vi "PH_PowerUnit_BaseClass.set modified data.vi"(0 "i ref in":refnum<vi>, 2 "i attribute":T1={"Constructor finished"=FALSE, "PU"={"In use"=FALSE, "Service ID in use"=-1, "GUI Ref"=refnum}, "Enabling"={"State"=0, "GUI Ref"=refnum}, "Timing"={"Last Shot"=0.0, "Time between Shots [Sec]"=30.0, "Waiting Time over?"=FALSE, "Service ID Waiting Time"=-1, "GUI Ref"=refnum, "Instance"={"Status"=0, "linked?"=FALSE, "GUI Ref"=refnum}}, "Sequencer"={"SM State"="N/A", "GUI Ref"=refnum, "linked"=FALSE}, "Subscribed Trendmssgs"=[], "PP PU"=enum."no Info", "Default Voltage (V)"=0.0, "GUI Refs"={"Delete Inst"=refnum, "State TO SM"=refnum, "State SM"=refnum, "Fire"=refnum}, "PSDB data"={"Shot Voltage [V]"=-1.0, "State TO SM"=enum.".", "Write 2 early"=FALSE}, "State TO SM"=enum."."} {"Subscribed Trendmssgs"."Shot Condition" items=["no info", "off/false/out", "on/true/in", "Failure", "Alarm", "Status 1", "Status 2", "Status 3"]; "Subscribed Trendmssgs"."Status" items=["no info", "off/false/out", "on/true/in", "Failure", "Alarm", "Status 1", "Status 2", "Status 3"]; "Timing"."Instance"."Status" items=["no info", "off/false/out", "on/true/in", "Failure", "Alarm", "Status 1", "Status 2", "Status 3"]; "Enabling"."State" items=["no info", "not disabled", "disabled"]}, 5 "error in (no error)":errorcluster) -> (14 "i ref out":refnum<vi>, 19 "error out":errorcluster)   [LabVIEW 2014, in "PH_PowerUnit_BaseClass.lvlib"]
doc: "Writes the data into the attribute of an object. Then, the attribute dara are unlocked using the \"release\" method. Prior to calling THIS method, the attribute data must have been locked using the methods \"lock\" or \"get data to modify\".\n\n\nLicense Agreement for this software:\n\nCopyright (C)\nGesellschaft für Schwerionenforschung, GSI\nPlanckstr. 1\n64291 Darmstadt\nGermany\n\nContact: D.Beck@gsi.de \n\nThis program is free software; you can redistribute it and/or modify it under the terms of the GNU General Public License as published by the Free Software Foundation; either version 2 of the license, or (at your option) any later version.\n\nThis program is distributed in the hope that it will be useful, but WITHOUT ANY WARRANTY; without even the implied warranty of MERCHANTABILITY or FITNESS FOR A PARTICULAR PURPOSE. See the GNU General License for more details (http://www.gnu.org).\n\nGesellschaft für Schwerionenforschung, GSI\nPlanckstr. 1, 64291 Darmstadt, Germany\nFor all questions and ideas contact: M.Richter@gsi.de, H.Brand@gsi.de or D.Beck@gsi.de.\nLast update: 17-JUN-2004"
uses:
  PH_PowerUnit_BaseClass.lvlib
  PH_PowerUnit_BaseClass.i attribute.ctl
  PH_SystemInformation/PH_SystemInformationEnabling State.ctl
  PH_StatusHandler/PH_StatusHandler.Status.ctl
  PH_PP_Common/PH_PP_Common.PUs.ctl
  PH_PowerUnit_BaseClass.GUI Refs.ctl
  PH_PowerUnit_BaseClass.SM States.ctl
  CS_Core/CSObj/CSObj.lvlib
  PH_SystemInformation/PH_SystemInformation.lvlib
  PH_StatusHandler/PH_StatusHandler.lvlib
  PH_PP_Common/PH_PP_Common.lvlib
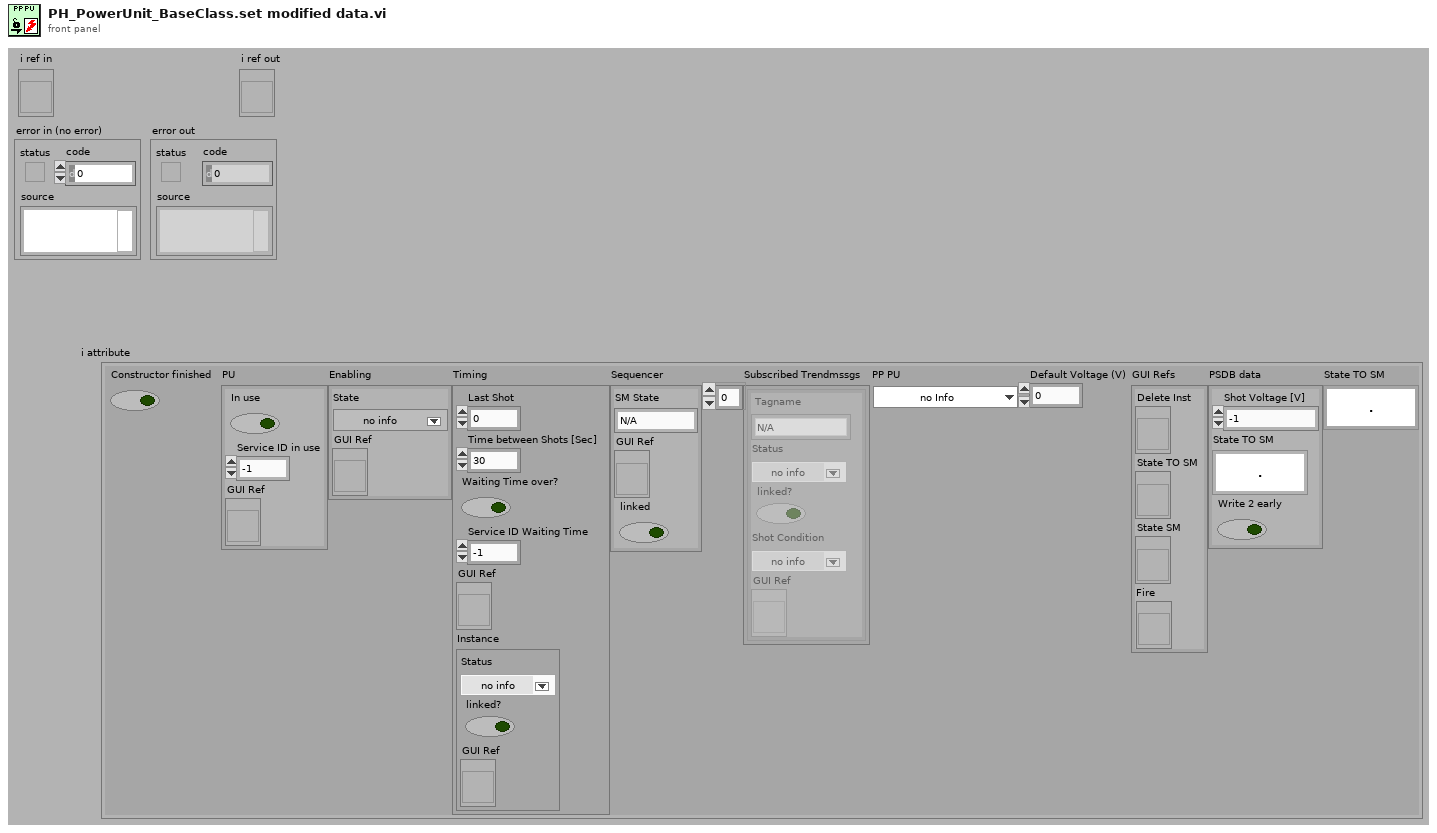
[diagram p1: front panel]
types:
  T1 = typedef "PH_PowerUnit_BaseClass.lvlib/PH_PowerUnit_BaseClass.i attribute.ctl" = cluster{"Constructor finished":bool, "PU":cluster{"In use":bool, "Service ID in use":i32, "GUI Ref":refnum<vi>}, "Enabling":cluster{"State":T2, "GUI Ref":refnum<vi>}, "Timing":cluster{"Last Shot":dbl, "Time between Shots [Sec]":dbl, "Waiting Time over?":bool, "Service ID Waiting Time":i32, "GUI Ref":refnum<vi>, "Instance":cluster{"Status":T3, "linked?":bool, "GUI Ref":refnum<vi>}}, "Sequencer":cluster{"SM State":string, "GUI Ref":refnum<vi>, "linked":bool}, "Subscribed Trendmssgs":cluster{"Tagname":string, "Status":T3, "linked?":bool, "Shot Condition":T3, "GUI Ref":refnum<vi>}[], "PP PU":T4, "Default Voltage (V)":dbl, "GUI Refs":T5, "PSDB data":cluster{"Shot Voltage [V]":dbl, "State TO SM":T6, "Write 2 early":bool}, "State TO SM":T6}
  T2 = typedef "PH_SystemInformation.lvlib/PH_SystemInformationEnabling State.ctl" = i32
  T3 = typedef "PH_StatusHandler.lvlib/PH_StatusHandler.Status.ctl" = i16
  T4 = typedef "PH_PP_Common.lvlib/PH_PP_Common.PUs.ctl" = enum16{"no Info", "PA-19mm-1", "PA-19mm-2", "PA-45mm-PILC", "PA-45mm-MAIN", "MA-PU-1", "MA-PU-2", "MA-PU-3", "MA-PU-4", "MA-PU-5", "MA-PU-6", "MA-FR", "MA-PILC", "PA-45mm-DP"}
  T5 = typedef "PH_PowerUnit_BaseClass.lvlib/PH_PowerUnit_BaseClass.GUI Refs.ctl" = cluster{"Delete Inst":refnum<vi>, "State TO SM":refnum<vi>, "State SM":refnum<vi>, "Fire":refnum<vi>}
  T6 = typedef "PH_PowerUnit_BaseClass.lvlib/PH_PowerUnit_BaseClass.SM States.ctl" = enum16{".", "Stand by", "Switch PU on", "Configure", "Set Default Voltage", "Set STANDBY", "Set READY", "Wait for Shot Cmd", "Open Dump Rods", "Open Ross Relais", "Close Ross Relais", "Switch PSU on", "Switch PSU off", "Charge", "Switch GD Channel on", "Close Dump Rods", "Rods-TO", "RR-TO", "PSU-TO", "Trigger-TO"}
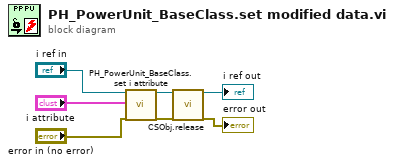
[diagram p0: block diagram]
diagram:
  n1 = call "PH_PowerUnit_BaseClass.set i attribute.vi"("i ref in"="i ref in", "i attribute"="i attribute", "error in (no error)"="error in (no error)") -> ("i ref out"=w4:refnum<vi>, "error out"=w3:errorcluster)  [unwired: 15 in]
  n2 = call "CSObj.release.vi"("i ref in"=w4, "error in (no error)"=w3) -> ("i ref out"=→"i ref out":refnum<vi>, "error out"=→"error out":errorcluster)  [unwired: 16 in]
